vi "BuildFileList.vi"() -> ()   [LabVIEW 2022 SP3]
panel:
  in  "Array":path[](array[path])=[path "\\\\Biomed-lab2\\d/Temp/Jeff Data/RRI Contrast Data/Point 1466", path "\\\\Biomed-lab2\\d/Temp/Jeff Data/RRI Contrast Data/Point 1470", path "\\\\Biomed-lab2\\d/Temp/Jeff Data/RRI Contrast Data/Point 1668"]
  out "String":string
  out "directory names":string[](array[string])
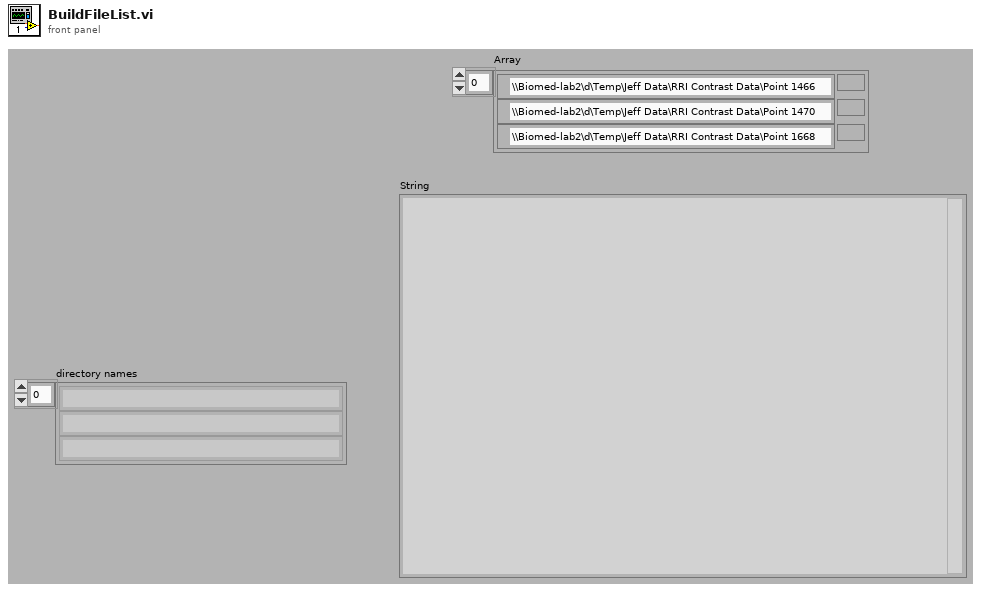
[diagram p1: front panel]
types:
  T1 = cluster{"Theraputic Freq (MHz)":sgl, "Time on (s)":sgl, "Therapy amplitude (mV)":sgl, "Lines Before":u16, "Lines After":u16}
  T2 = cluster{"RF file name":string, "RF file att":string, "RF cal file name":string, "RF cal file att":string}
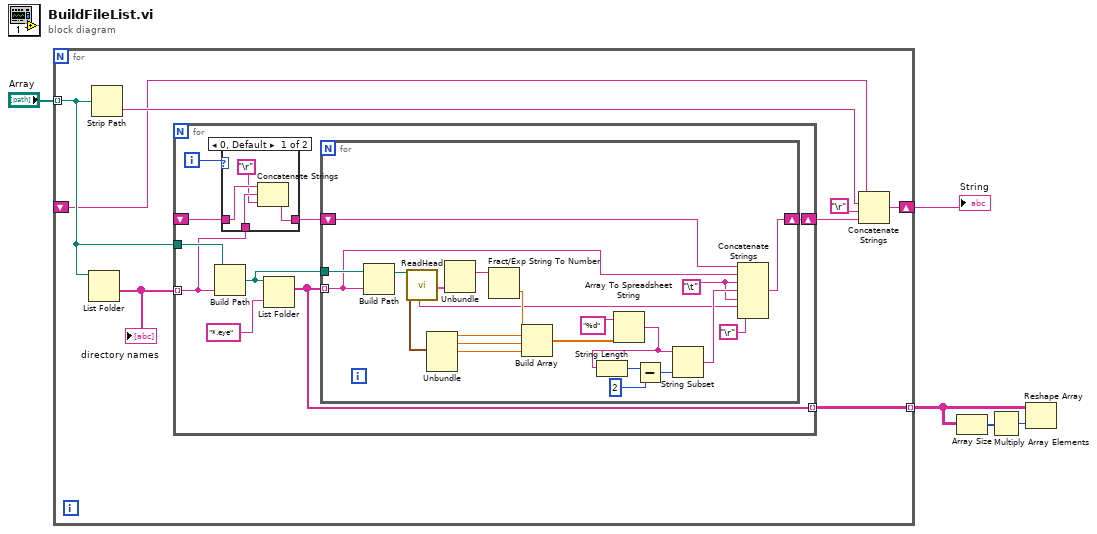
[diagram p0: block diagram]
diagram:
  n1 = for {
    tunnel: "Array" -> [w9] mode=indexing
    shift-right: [w8] -> w4
    shift-left: _ -> [w7]
    tunnel: [w6] -> w1 mode=indexing
    n2 = List Folder(path=w9) -> (folder names=w13:string[])  [unwired: 1 in, 5 out]
    "directory names" <- w13
    n3 = Strip Path(path=w9) -> (name=w11:string)  [unwired: 1 out]
    n4 = for {
      tunnel: w13 -> [w14] mode=indexing
      tunnel: w9 -> [w22]
      tunnel: [w21] -> w6 mode=indexing
      shift-right: [w18] -> w12
      shift-left: _ -> [w16]
      i -> [w17]
      n5 = Build Path(base path=w22, name or relative path=w14) -> (appended path=w20:path)
      n6 = case shown="0, Default" w17 {
        tunnel: [w25 w27] -> w15
        tunnel: w16 -> [w26 w27]
        tunnel: w14 -> [w24 _]
        frame 0, Default {
          n7 = Concatenate Strings(w26, w24, "\r") -> (w25:string)
        }
        frame 1 {
        }
      }
      n8 = List Folder(path=w20, pattern="*.eye") -> (filenames=w21:string[])  [unwired: 1 in, 4 out]
      n9 = for {
        tunnel: w21 -> [w37] mode=indexing
        tunnel: w20 -> [w49]
        shift-right: [w38] -> w18
        shift-left: w15 -> [w36]
        w30 = "\t"
        n10 = Build Path(base path=w49, name or relative path=w37) -> (appended path=w48:path)
        n11 = call "ReadHead.vi"("new file path"=w48) -> ("Therapy Parameters"=w47:T1, "Comment"=w29:string, "RF Info"=w43:T2)  [unwired: 16 out]
        n12 = Unbundle(w47) -> ("Theraputic Freq (MHz)"=w46:sgl, "Time on (s)"=w45:sgl, "Therapy amplitude (mV)"=w44:sgl)  [unwired: 2 out]
        n13 = Unbundle(w43) -> ("RF file att"=w42:string)  [unwired: 3 out]
        n14 = Fract/Exp String To Number(string=w42) -> (number=w41:dbl)  [unwired: 4 out]
        n15 = Build Array(w41, w46, w45, w44) -> (w40:dbl[])
        n16 = Array To Spreadsheet String(array=w40, 3:"%d" ("format string")) -> (spreadsheet string=w32:string)  [unwired: 1 out]
        n17 = String Length(string=w32) -> (length=w35:i32)
        n18 = Subtract(x=w35, y=2) -> (x-y=w34:i32)
        n19 = String Subset(string=w32, length (rest)=w34) -> (substring=w31:string)  [unwired: 1 out]
        n20 = Concatenate Strings(w36, w37, w30, w31, w30, w29, "\r") -> (w38:string)
      }
    }
    n21 = Concatenate Strings(w7, w11, "\r", w12) -> (w8:string)
  }
  "String" <- w4
  n22 = Array Size(array=w1) -> (size(s)=w2:i32[])
  n23 = Multiply Array Elements(1:w2) -> (0:w3:i32)
  n24 = Reshape Array(w1, w3) -> ()  [unwired: 1 out]
